vi "Set Clock (Calendar).vi"(0 "VISA resource name":refnum<visa-resource-name>, 1 "Minute (0)":i32, 2 "Hour (0)":i32, 5 "Second (0)":i32, 7 "Day (1)":i32=1, 9 "Month (1: January)":u32(ring)=1 items=["", "January", "February", "March", "April", "May", "June", "July", "August", "Septemeber", "October", "Novemeber", "December"], 11 "error in (no error)":errorcluster, 12 "Year (2002)":i32=2002) -> (4 "VISA resource name out":refnum<visa-resource-name>, 15 "error out":errorcluster)   [LabVIEW 2014, in "Fluke 5XXX Series Multicalibrators.lvlib"]
doc: "This VI configures the instrument's internal clock and calendar.\n\nNotes:\n\n(1) This VI is available only for instrument models 5520A, 5700A and 5720A.\n\n(2) You will be unable to set the clock (calendar) if the rear panel CALIBRATION switch is in the ENABLE position."
uses:
  Fluke 5XXX Series Multicalibrators.lvlib
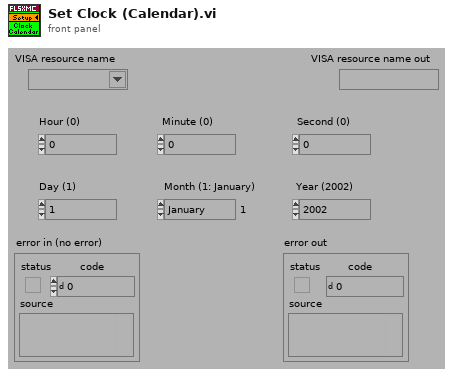
[diagram p1: front panel]
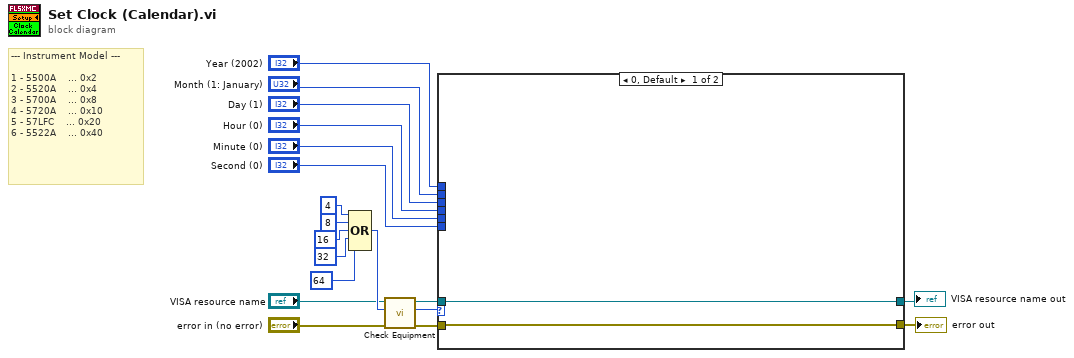
[diagram p0: block diagram]
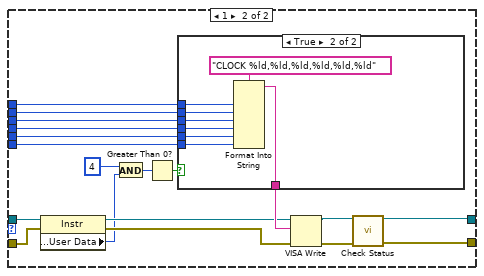
[diagram p2: hidden frame]
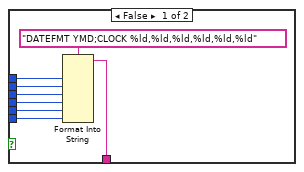
[diagram p3: hidden frame]
diagram:
  # "--- Instrument Model ---\n\n1 - 5500A    ... 0x2\n2 - 5520A    ... 0x4\n3 - 5700A    ... 0x8\n4 - 5720A    ... 0x10\n5 - 57LFC    ... 0x20\n6 - 5522A    ... 0x40"
  n1 = Compound Arithmetic op=OR(4 ("Numeric"), 8 ("Numeric"), 16 ("Numeric"), 32 ("Numeric"), 64 ("Numeric")) -> (w13:i32)
  n2 = call "Check Equipment.vi"("error in (no error)"="error in (no error)", "Bit Mask"=w13, "VISA resource name"="VISA resource name") -> ("error out"=w16:errorcluster, "Present?"=w14:u32, "VISA resource name out"=w15:refnum<visa-resource-name>)  [unwired: 6 in]
  n3 = case shown="0, Default" w14 {
    tunnel: [w20 w37] -> w11
    tunnel: w16 -> [w21 w27]
    tunnel: w15 -> [w20 w29]
    tunnel: [w21 w40] -> w12
    tunnel: "Year (2002)" -> [_ w35]
    tunnel: "Month (1: January)" -> [_ w34]
    tunnel: "Day (1)" -> [_ w33]
    tunnel: "Hour (0)" -> [_ w32]
    tunnel: "Minute (0)" -> [_ w31]
    tunnel: "Second (0)" -> [_ w30]
    frame 0, Default {
    }
    frame 1 {
      n4 = property class="Instr"(reference=w29, error in=w27) -> (reference out=w28:refnum<visa-resource-name>, error out=w26:errorcluster, "General Settings:User Data"=w25:u32)
      n5 = And(x=u32 4 ("Numeric"), y=w25) -> (x .and. y?=w23:u32)
      n6 = Greater Than 0?(x=w23) -> (x > 0?=w22:bool)
      n7 = case shown="True" w22 {
        tunnel: [w47 w55] -> w36
        tunnel: w35 -> [w46 w54]
        tunnel: w34 -> [w45 w53]
        tunnel: w33 -> [w44 w52]
        tunnel: w32 -> [w43 w51]
        tunnel: w31 -> [w42 w50]
        tunnel: w30 -> [w41 w49]
        frame False {
          n8 = Format Into String(format string="DATEFMT YMD;CLOCK %ld,%ld,%ld,%ld,%ld,%ld", w46, w45, w44, w43, w42, w41) -> (resulting string=w47:string)  [unwired: 2 in, 1 out]
        }
        frame True {
          n9 = Format Into String(format string="CLOCK %ld,%ld,%ld,%ld,%ld,%ld", w54, w53, w52, w51, w50, w49) -> (resulting string=w55:string)  [unwired: 2 in, 1 out]
        }
      }
      n10 = VISA Write(VISA resource name=w28, write buffer=w36, error in (no error)=w26) -> (VISA resource name out=w38:refnum<visa-resource-name>, error out=w39:errorcluster)  [unwired: 1 out]
      n11 = call "Check Status.vi"("VISA resource name"=w38, "error in (no error)"=w39) -> ("VISA resource name out"=w37:refnum<visa-resource-name>, "error out"=w40:errorcluster)  [unwired: 12 in]
    }
  }
  "VISA resource name out" <- w11
  "error out" <- w12
